vi "AverageSampleHold_slow.vi"(8 "Previous Average":i32, 9 "Input Value":i32) -> (2 "Output New Average":i32)   [LabVIEW 2013]
uses:
  <vilib>/rvi/FIFO/Fifo_Resource/nirvififoEmulationReadFpgaImpl.vi
  <vilib>/rvi/DataTransferAndStorage/Container/Common/niFpgaContainerGetUniqueNameForEmu.vi
  <vilib>/rvi/FIFO/Fifo_Resource/nirvififoEmulationWriteFpgaImpl.vi
  <vilib>/rvi/DataTransferAndStorage/Container/XNode/niFpgaContainer.xnode
  <vilib>/rvi/FIFO/Fifo_Resource/nirvififoEmulationRead.vi
  <vilib>/rvi/FIFO/Fifo_Resource/nirvififoEmulationWrite.vi
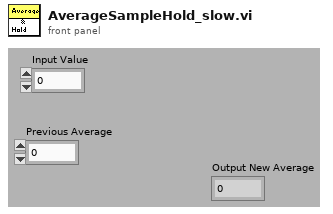
[diagram p1: front panel]
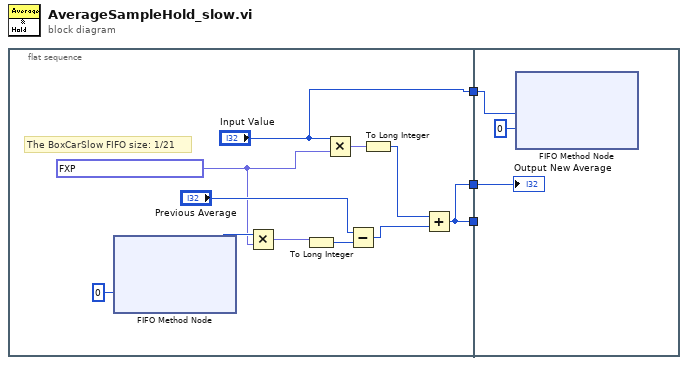
[diagram p0: block diagram]
diagram:
  n1 = flat-sequence {
    tunnel: ["Input Value"] -> w3
    tunnel: [w10] -> w2
    tunnel: [w10] -> w1
    tunnel: w3 -> [w17]
    tunnel: w2 -> [_]
    tunnel: w1 -> [w16]
    frame #0 {
      w7 = fxp<+,19,-4> 0.04762005805969238 ("y")
      # "The BoxCarSlow FIFO size: 1/21"
      n2 = xnode ("FIFO Method Node")("Timeout"=0) -> ("Element"=w8:i32)  [unwired: 1 in, 2 out]
      n3 = Multiply(x=w8, y=w7) -> (x*y=w5:fxp<+/-,51,28>)
      n4 = To Long Integer(number=w5) -> (32bit integer=w6:i32)
      n5 = Multiply(x="Input Value", y=w7) -> (x*y=w12:fxp<+/-,51,28>)
      n6 = Subtract(x="Previous Average", y=w6) -> (x-y=w13:i32)
      n7 = To Long Integer(number=w12) -> (32bit integer=w11:i32)
      n8 = Add(x=w11, y=w13) -> (x+y=w10:i32)
    }
    frame #1 {
      n9 = xnode ("FIFO Method Node")("Element"=w17, "Timeout"=0) -> ()  [unwired: 1 in, 2 out]
      "Output New Average" <- w16
    }
  }
